vi "Phasor Cosine-Sine Complex Vector.vi"(6 "Use Gate Center":bool, 8 "Phasor Frequency":dbl[unit], 9 "Elementary Gate Separation":dbl[unit], 10 "Step":i32, 11 "# Gates":i32) -> (3 "e^j w t_i Vector":csg[](array[numeric]) format="%_3e")   [LabVIEW 2021, in "Phasor.lvlib"]
uses:
  Phasor.lvlib
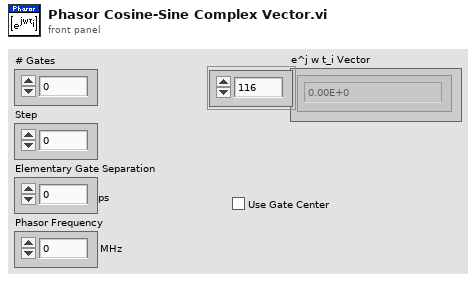
[diagram p1: front panel]
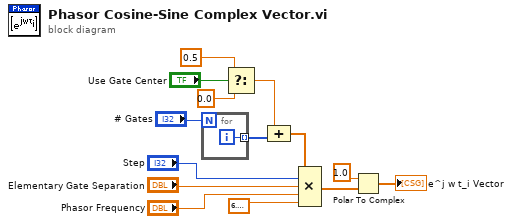
[diagram p0: block diagram]
diagram:
  n1 = for {
    N: "# Gates" -> [_]
    tunnel: [w15] -> w7 mode=indexing
    i -> [w15]
  }
  n2 = Select(t=0.5 ("start"), s="Use Gate Center", f=0.0) -> (s? t:f=w2:dbl)
  n3 = Compound Arithmetic op=unknown(w2, w7) -> (w5:dbl[])
  n4 = Compound Arithmetic op=MULTIPLY(w5, "Step", "Elementary Gate Separation", "Phasor Frequency", 6.283185307179586) -> (w6:dbl[])
  n5 = Polar To Complex(1:w6, 2:1.0 ("start")) -> (0:→"e^j w t_i Vector":cdb[])
